vi "Float to Go Format.vi"(11 "Float Value":dbl format="%#_12f") -> (3 "Go Format":string)   [LabVIEW 2020]
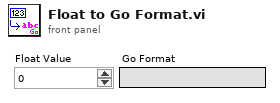
[diagram p1: front panel]
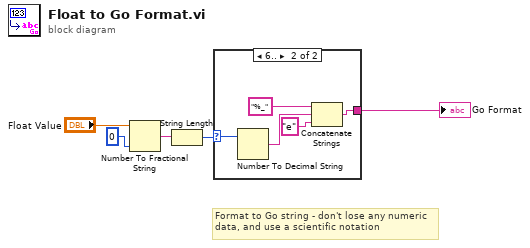
[diagram p0: block diagram]
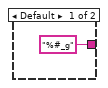
[diagram p2: hidden frame]
diagram:
  # "Format to Go string - don't lose any numeric data, and use a scientific notation"
  n1 = Number To Fractional String(number="Float Value", precision (6)=i16 0) -> (F-format string=w2:string)  [unwired: 2 in]
  n2 = String Length(string=w2) -> (length=w3:i32)
  n3 = case shown="6.." w3 {
    selector: w3 -> [_ w11]
    tunnel: ["%#_g" w8] -> w5
    frame Default {
    }
    frame 6.. {
      n4 = Number To Decimal String(number=w11) -> (decimal integer string=w9:string)  [unwired: 1 in]
      n5 = Concatenate Strings("%_" ("string"), w9, "e" ("string")) -> (w8:string)
    }
  }
  "Go Format" <- w5
